vi "温度湿度监测界面.vi"() -> ()   [LabVIEW 2016, in "环境动力监测库.lvlib"]
panel:
  out "x+1":u32
  in  "解除告警":bool
  out "告警内容":string
  in  "高温告警启用":bool
  out "湿度显示":dbl=21.0 format="%.2f %%"
  out "湿度":dbl(graph)
  out "温度显示":dbl=21.0 format="%.2f ℃"
  out "温度":dbl(graph)
  in  "湿度下限告警点":dbl
  in  "湿度上限告警点":dbl
  in  "室温下限告警点":dbl
  in  "室温上限告警点":dbl
  # "温湿度监测"
  # "%"
  # "℃"
  # "%"
  # "℃"
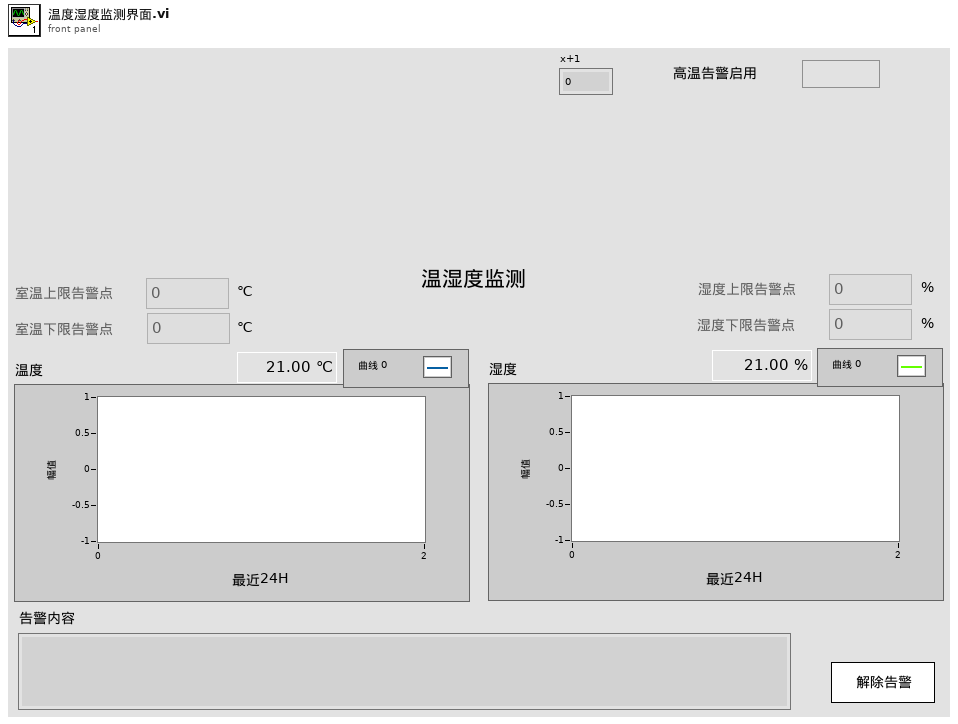
[diagram p1: front panel]
types:
  T1 = enum16{"报警状态监测", "报警确认", "仪器断电", "市电断电", "工控机关机", "取消告警", "结束"}
  T2 = cluster{"漏水监测输出":cluster{"漏水监测告警":bool, "告警内容":string}, "门禁监测输出":cluster{"门禁监测告警":bool, "告警内容":string}, "门禁监测输出2":cluster{"门禁监测告警":bool, "告警内容":string}, "温湿度监测输出":cluster{"温湿度监测告警":bool, "告警内容":string}, "烟雾监测输出":cluster{"烟雾监测告警":bool, "告警内容":string}, "空调监测输出":cluster{"空调监测告警":bool, "告警内容":string}, "自动重合闸输出":cluster{"自动重合闸告警":bool, "告警内容":string}, "红外入侵输出":cluster{"红外入侵告警":bool, "告警内容":string}, "振动输出":cluster{"振动告警":bool, "告警内容":string}, "UPS输出":cluster{"UPS告警":bool, "告警内容":string}, "蓄电池输出":cluster{"蓄电池告警":bool, "告警内容":string}, "蓄电池输出2":cluster{"蓄电池告警":bool, "告警内容":string}, "GPS输出":cluster{"定位告警":bool, "告警内容":string}, "北斗输出":cluster{"定位告警":bool, "告警内容":string}, "气象输出":cluster{"气象告警":bool, "告警内容":string}}
  T3 = cluster{"漏水监测配置":cluster{"监测项描述:输出":string, "端口:":enum16{"AI0", "AI1", "AI2", "AI3", "AI4", "DI0", "DI1", "DI2", "DI3", "DI4", "DO0", "DO1", "DO2", "DO3", "DO4", "X0", "X1", "X2", "X3", "X4", "X5", "X6", "X7", "X8", "X9", "X10", "X11", "X12", "X13", "X14", "X15", "X16", "X17", "X18", "X19", "X20", "X21", "X22", "X23"}, "告警参数:":enum32{"禁用告警", "闭合告警", "断开告警"}, "传感器型号:":enum16{"PLC", "ZLAN", "ART"}, "声光告警启用":bool}, "门禁开关监测配置":cluster{"监测项描述:输出":string, "端口:":enum16{"AI0", "AI1", "AI2", "AI3", "AI4", "DI0", "DI1", "DI2", "DI3", "DI4", "DO0", "DO1", "DO2", "DO3", "DO4", "X0", "X1", "X2", "X3", "X4", "X5", "X6", "X7", "X8", "X9", "X10", "X11", "X12", "X13", "X14", "X15", "X16", "X17", "X18", "X19", "X20", "X21", "X22", "X23"}, "告警参数:":enum32{"禁用告警", "闭合告警", "断开告警"}, "传感器型号:":enum16{"PLC", "ZLAN", "ART"}, "声光告警启用":bool}, "门禁开关监测配置2":cluster{"监测项描述:输出":string, "端口:":enum16{"AI0", "AI1", "AI2", "AI3", "AI4", "DI0", "DI1", "DI2", "DI3", "DI4", "DO0", "DO1", "DO2", "DO3", "DO4", "X0", "X1", "X2", "X3", "X4", "X5", "X6", "X7", "X8", "X9", "X10", "X11", "X12", "X13", "X14", "X15", "X16", "X17", "X18", "X19", "X20", "X21", "X22", "X23"}, "告警参数:":enum32{"禁用告警", "闭合告警", "断开告警"}, "传感器型号:":enum16{"PLC", "ZLAN", "ART"}, "声光告警启用":bool}, "温湿度监测配置":cluster{"监测项描述:输出":string, "端口:":enum16{"AI0", "AI1", "AI2", "AI3", "AI4", "DI0", "DI1", "DI2", "DI3", "DI4", "DO0", "DO1", "DO2", "DO3", "DO4", "X0", "X1", "X2", "X3", "X4", "X5", "X6", "X7", "X8", "X9", "X10", "X11", "X12", "X13", "X14", "X15", "X16", "X17", "X18", "X19", "X20", "X21", "X22", "X23"}, "告警参数:":enum32{"禁用告警", "闭合告警", "断开告警"}, "传感器型号:":enum16{"PLC", "ZLAN", "ART"}, "声光告警启用":bool}, "烟雾监测配置":cluster{"监测项描述:输出":string, "端口:":enum16{"AI0", "AI1", "AI2", "AI3", "AI4", "DI0", "DI1", "DI2", "DI3", "DI4", "DO0", "DO1", "DO2", "DO3", "DO4", "X0", "X1", "X2", "X3", "X4", "X5", "X6", "X7", "X8", "X9", "X10", "X11", "X12", "X13", "X14", "X15", "X16", "X17", "X18", "X19", "X20", "X21", "X22", "X23"}, "告警参数:":enum32{"禁用告警", "闭合告警", "断开告警"}, "传感器型号:":enum16{"PLC", "ZLAN", "ART"}, "声光告警启用":bool}, "冰箱监测配置":cluster{"监测项描述:输出":string, "端口:":enum16{"AI0", "AI1", "AI2", "AI3", "AI4", "DI0", "DI1", "DI2", "DI3", "DI4", "DO0", "DO1", "DO2", "DO3", "DO4", "X0", "X1", "X2", "X3", "X4", "X5", "X6", "X7", "X8", "X9", "X10", "X11", "X12", "X13", "X14", "X15", "X16", "X17", "X18", "X19", "X20", "X21", "X22", "X23"}, "告警参数:":enum32{"禁用告警", "闭合告警", "断开告警"}, "传感器型号:":enum16{"PLC", "ZLAN", "ART"}, "声光告警启用":bool}, "排气扇监测配置":cluster{"监测项描述:输出":string, "端口:":enum16{"AI0", "AI1", "AI2", "AI3", "AI4", "DI0", "DI1", "DI2", "DI3", "DI4", "DO0", "DO1", "DO2", "DO3", "DO4", "X0", "X1", "X2", "X3", "X4", "X5", "X6", "X7", "X8", "X9", "X10", "X11", "X12", "X13", "X14", "X15", "X16", "X17", "X18", "X19", "X20", "X21", "X22", "X23"}, "告警参数:":enum32{"禁用告警", "闭合告警", "断开告警"}, "传感器型号:":enum16{"PLC", "ZLAN", "ART"}, "声光告警启用":bool}, "红外入侵监测配置":cluster{"监测项描述:输出":string, "端口:":enum16{"AI0", "AI1", "AI2", "AI3", "AI4", "DI0", "DI1", "DI2", "DI3", "DI4", "DO0", "DO1", "DO2", "DO3", "DO4", "X0", "X1", "X2", "X3", "X4", "X5", "X6", "X7", "X8", "X9", "X10", "X11", "X12", "X13", "X14", "X15", "X16", "X17", "X18", "X19", "X20", "X21", "X22", "X23"}, "告警参数:":enum32{"禁用告警", "闭合告警", "断开告警"}, "传感器型号:":enum16{"PLC", "ZLAN", "ART"}, "声光告警启用":bool}, "振动监测配置":cluster{"监测项描述:输出":string, "端口:":enum16{"AI0", "AI1", "AI2", "AI3", "AI4", "DI0", "DI1", "DI2", "DI3", "DI4", "DO0", "DO1", "DO2", "DO3", "DO4", "X0", "X1", "X2", "X3", "X4", "X5", "X6", "X7", "X8", "X9", "X10", "X11", "X12", "X13", "X14", "X15", "X16", "X17", "X18", "X19", "X20", "X21", "X22", "X23"}, "告警参数:":enum32{"禁用告警", "闭合告警", "断开告警"}, "传感器型号:":enum16{"PLC", "ZLAN", "ART"}, "声光告警启用":bool}}
  T4 = cluster{"监测项描述:输出":string, "端口:":enum16{"AI0", "AI1", "AI2", "AI3", "AI4", "DI0", "DI1", "DI2", "DI3", "DI4", "DO0", "DO1", "DO2", "DO3", "DO4", "X0", "X1", "X2", "X3", "X4", "X5", "X6", "X7", "X8", "X9", "X10", "X11", "X12", "X13", "X14", "X15", "X16", "X17", "X18", "X19", "X20", "X21", "X22", "X23"}, "告警参数:":enum32{"禁用告警", "闭合告警", "断开告警"}, "传感器型号:":enum16{"PLC", "ZLAN", "ART"}, "声光告警启用":bool}
  T5 = enum16{"AI0", "AI1", "AI2", "AI3", "AI4", "DI0", "DI1", "DI2", "DI3", "DI4", "DO0", "DO1", "DO2", "DO3", "DO4", "X0", "X1", "X2", "X3", "X4", "X5", "X6", "X7", "X8", "X9", "X10", "X11", "X12", "X13", "X14", "X15", "X16", "X17", "X18", "X19", "X20", "X21", "X22", "X23"}
  T6 = cluster{"市电监测":bool, "用水量监测":bool, "烟雾监测":bool, "温度湿度":bool, "振动监测":bool, "红外入侵监测":bool, "漏水监测":bool, "门禁开关监测":bool, "门禁开关监测2":bool, "视频监测":bool, "UPS监测":bool, "空调监测":bool, "冰箱监测":bool, "排气扇监测":bool, "蓄电池监测":bool, "蓄电池监测2":bool, "GPS监测":bool, "北斗监测":bool, "气象监测":bool, "智能门禁监测":bool}
  T7 = cluster{"状态":cluster{"R0":i16, "R1":i16, "R2":i16, "R3":i16, "R4":i16, "R5":i16, "R6":i16, "R7":i16, "R8":i16, "R9":i16, "R10":i16, "R11":i16, "R12":i16, "R13":i16, "R14":i16, "R15":i16, "R16":i16, "R17":i16, "R18":i16, "R19":i16, "R20":i16, "R21":i16, "R22":i16, "R23":i16, "R24":i16, "R25":i16, "R26":i16, "R27":i16, "R28":i16, "R29":i16, "R30":i16, "R31":i16, "R32":i16, "R33":i16, "R34":i16, "R35":i16, "R36":i16, "R37":i16, "R38":i16, "R39":i16}, "输入状态":bool[], "输出状态":bool[], "参数设置":cluster{"R100":i16, "R101":i16, "R102":i16, "R103":i16, "R104":i16, "R105":i16, "R106":i16, "R107":i16, "R108":i16, "R109":i16, "R110":i16, "R111":i16, "R112":i16, "R113":i16, "R114":i16, "R115":i16, "R116":i16, "R117":i16, "R118":i16, "R119":i16, "R120":i16, "R121":i16, "R122":i16, "R123":i16}, "转换值":cluster{"AD0":sgl, "AD1":sgl, "AD2":sgl, "AD3":sgl, "AD4":sgl, "AD5":sgl}}
  T8 = cluster{"型号选择":enum16{"黑盾", "英维克", "仁科测控RS-KTC-N01"}, "MB session in":refnum<class "MB_Master.lvclass">, "英维克空调寄存器":u16[], "通讯状态":bool, "PORT":string, "IP":string, "Slave ID ":u8, "Serial Config":cluster{"baud rate (bps)":u32, "stop bits":u16, "parity":u16, "flow control":u16, "timeout":u32, "retries":i32}, "VISA Resource":refnum<visa-resource-name>, "MB通信方式选择":enum16{"串口", "TCP"}}
  T9 = cluster{"温湿度解析":cluster{"湿度":dbl, "温度":dbl}, "传感器状态输出":cluster{"第一路电流A":u16, "第二路电流A":u16, "空调控制模式":enum16{"远程", "自动"}, "蜂鸣器和继电器报警输出状态":enum16{"正常", "报警"}, "秒数高16位":u16, "秒数低16位":u16}, "告警状态":cluster{"第一路开关机失败":bool, "第二路开关机失败":bool, "温度超上限报警":bool, "温度超下限报警":bool}, "运行状态":cluster{"第一路空调运行状态":enum16{"停止", "制冷", "制热", "未知"}, "第二路空调运行状态":enum16{"停止", "制冷", "制热", "未知"}}}
  T10 = cluster{"状态":cluster{"R0":i16, "R1":i16, "R2":i16, "R3":i16, "R4":i16, "R5":i16, "R6":i16, "R7":i16, "R8":i16, "R9":i16, "R10":i16, "R11":i16, "R12":i16, "R13":i16, "R14":i16, "R15":i16, "R16":i16, "R17":i16, "R18":i16, "R19":i16, "R20":i16, "R21":i16, "R22":i16, "R23":i16, "R24":i16, "R25":i16, "R26":i16, "R27":i16, "R28":i16, "R29":i16, "R30":i16, "R31":i16, "R32":i16, "R33":i16, "R34":i16, "R35":i16, "R36":i16, "R37":i16, "R38":i16, "R39":i16, "R40":i16, "R41":i16, "R42":i16, "R43":i16, "R44":i16, "R45":i16, "R46":i16, "R47":i16, "R48":i16, "R49":i16, "R50":i16, "R51":i16, "R52":i16, "R53":i16, "R54":i16, "R55":i16, "R56":i16, "R57":i16, "R58":i16, "R59":i16, "R60":i16, "R61":i16, "R62":i16, "R63":i16, "R64":i16, "R65":i16, "R66":i16, "R67":i16, "R68":i16, "R69":i16}, "输入状态":bool[], "输出状态":bool[], "报警簇":bool[], "参数设置":cluster{"R100":i16, "R101":i16, "R102":i16, "R103":i16, "R104":i16, "R105":i16, "R106":i16, "R107":i16, "R108":i16, "R109":i16, "R110":i16, "R111":i16, "R112":i16, "R113":i16, "R114":i16, "R115":i16, "R116":i16, "R117":i16, "R118":i16, "R119":i16, "R120":i16, "R121":i16, "R122":i16, "R123":i16, "R124":i16}, "转换值":cluster{"AD0":sgl, "AD1":sgl, "AD2":sgl, "AD3":sgl, "AD4":sgl, "AD5":sgl}, "看门狗启用":bool, "氨氮模块名称":string, "总磷模块名称":string, "采配水模块类型":enum16{"V1", "V2", "V3", "V4", "室内V1", "室内V2"}}
  T11 = cluster{"AD0":dbl, "AD1":dbl, "AD2":dbl, "AD3":dbl, "AD4":dbl, "AD5":dbl, "AD6":dbl, "AD7":dbl}
  T12 = cluster{"命令":string, cluster{"starting address":u16, "holding register value":u16}}
  T13 = cluster{"温湿度":cluster{"状态":bool, "温度:":sgl, "湿度:":sgl, "详情  ":bool}, "空调":cluster{"状态":bool, "机柜温度:":sgl, "压缩机:":enum16{"停止", "运行"}, "电加热:":enum16{"停止", "运行"}, "详情  ":bool}, "排气扇":cluster{"排气扇":bool, "详情  ":bool}, "冰箱":cluster{"冰箱":bool, "详情  ":bool}}
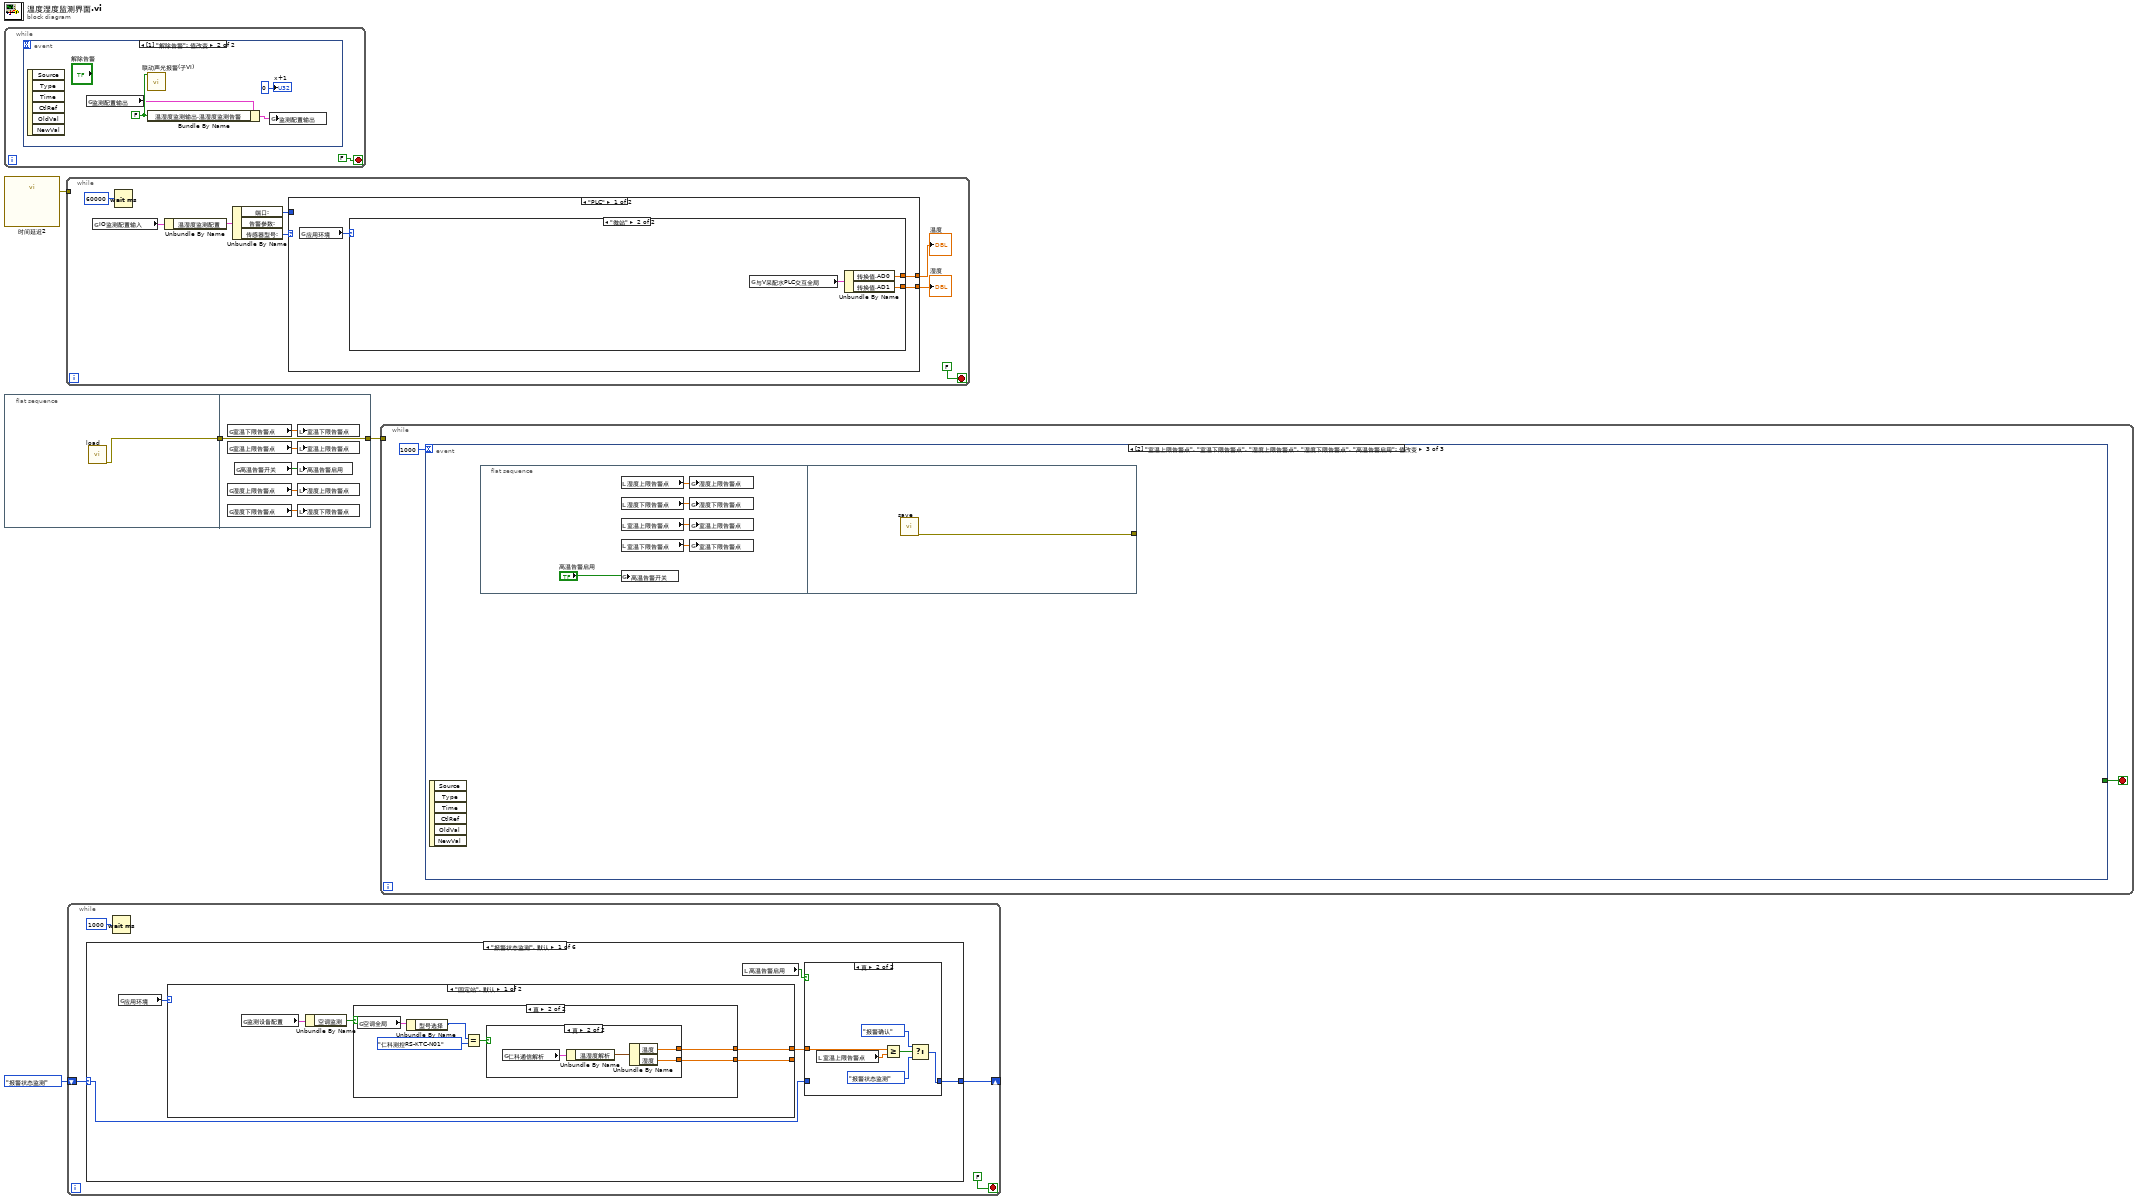
[diagram p0: block diagram]
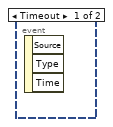
[diagram p2: hidden frame]
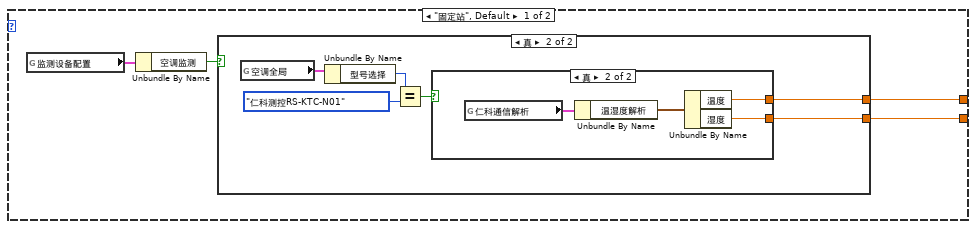
[diagram p3: hidden frame]
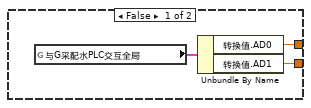
[diagram p4: hidden frame]
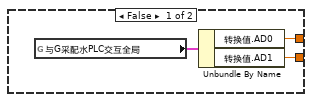
[diagram p5: hidden frame]
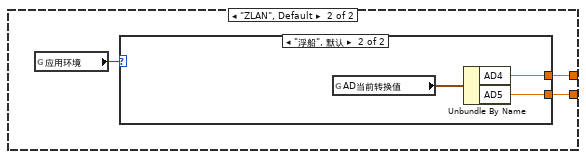
[diagram p6: hidden frame]
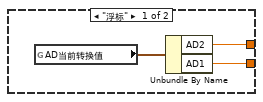
[diagram p7: hidden frame]
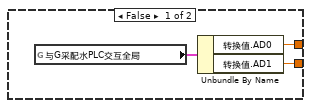
[diagram p8: hidden frame]
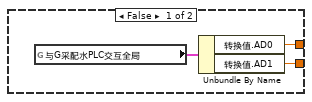
[diagram p9: hidden frame]
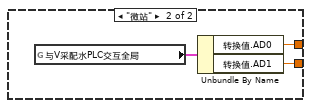
[diagram p10: hidden frame]
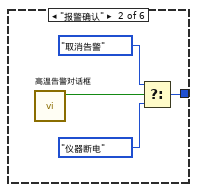
[diagram p12: hidden frame]
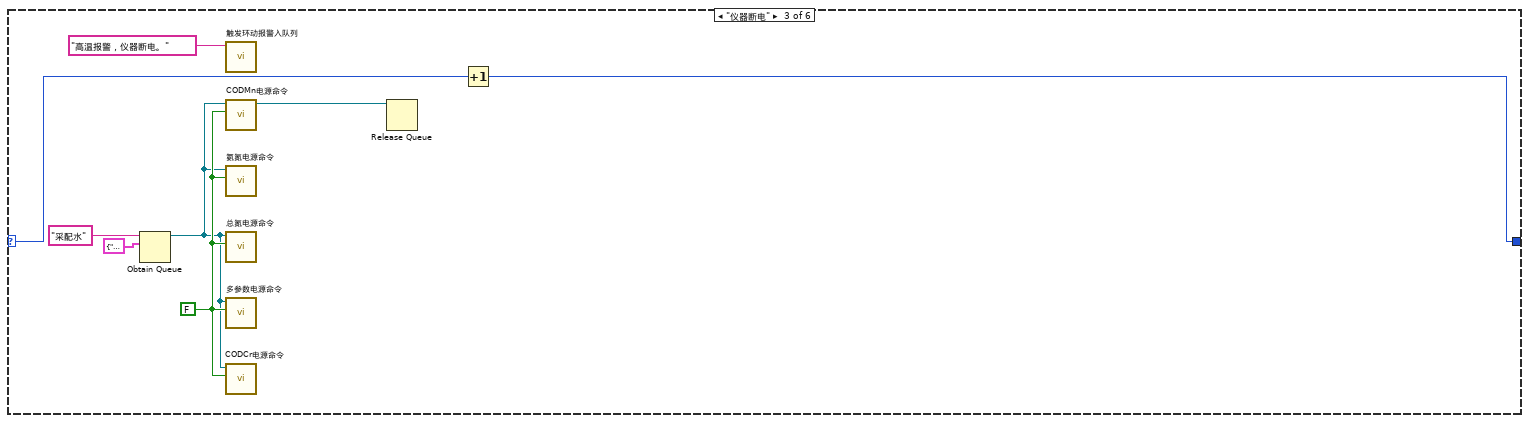
[diagram p13: hidden frame]
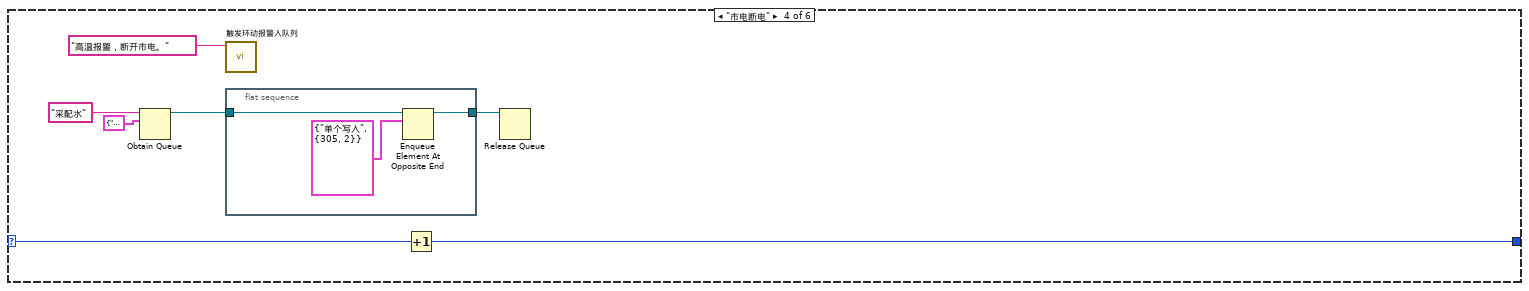
[diagram p14: hidden frame]
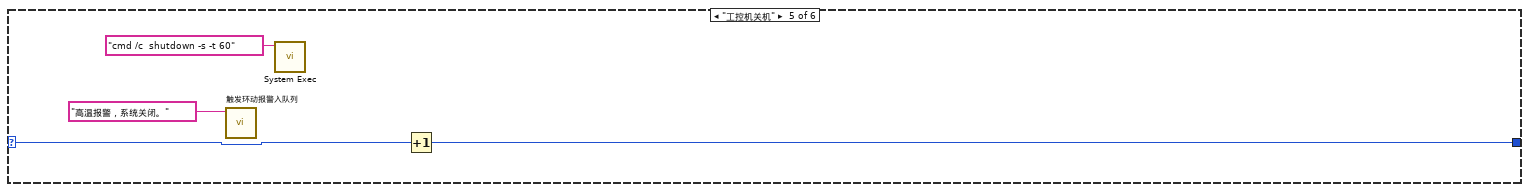
[diagram p15: hidden frame]
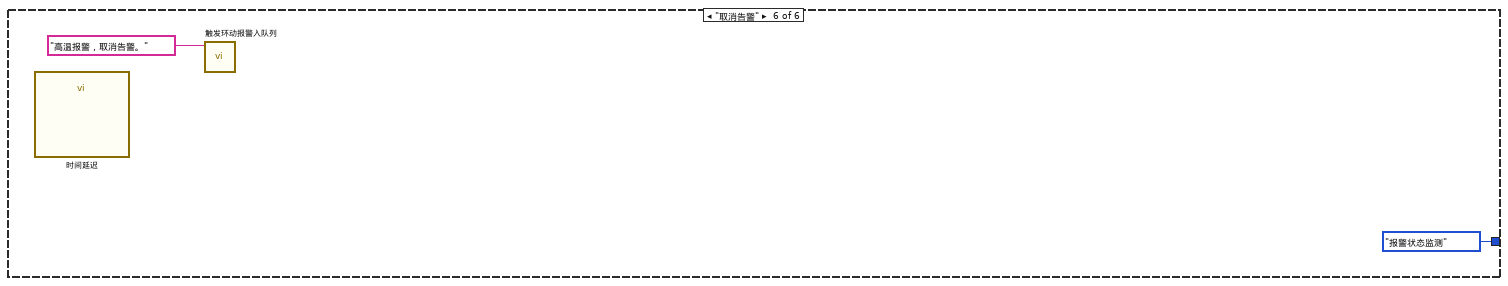
[diagram p16: hidden frame]
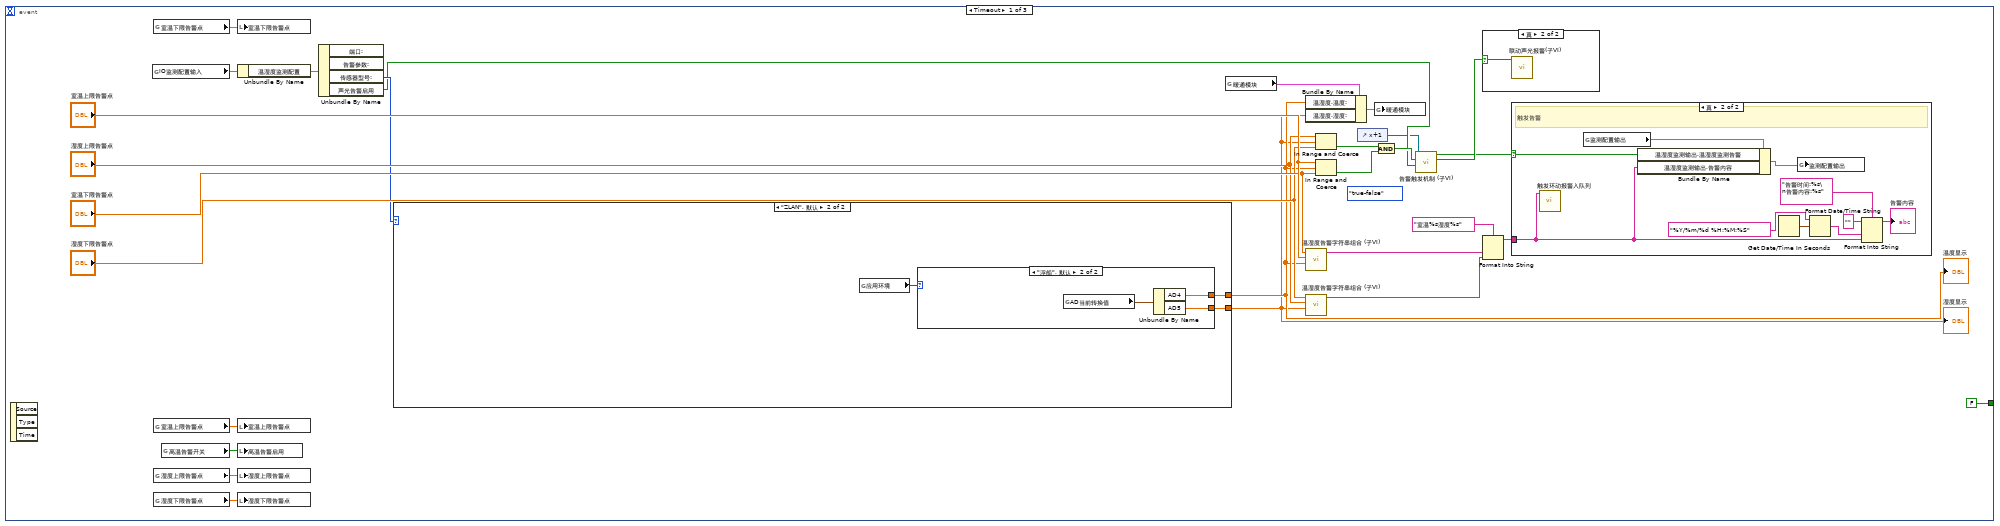
[diagram p17: hidden frame]
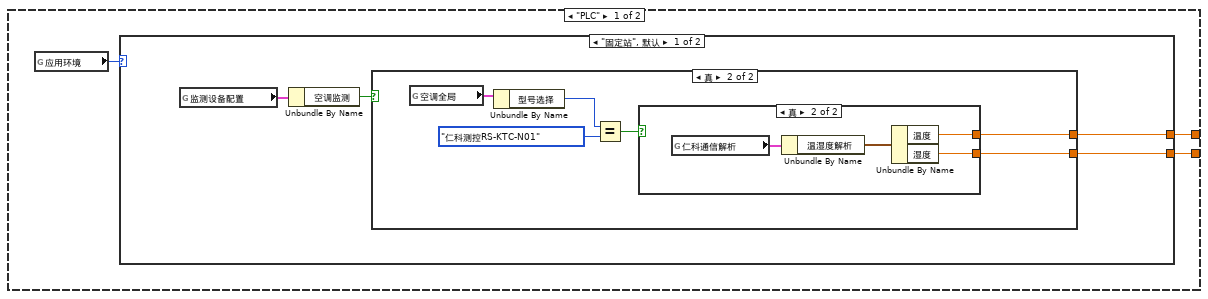
[diagram p19: hidden frame]
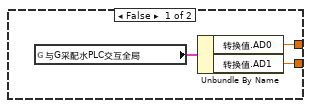
[diagram p20: hidden frame]
diagram:
  n1 = while {
    stop <- FALSE stop-if-true
    n2 = event shown="[1] \"解除告警\": 值改变" {
      selector: _ -> [_ _]
      dyn-events: _ -> [_ _]
      timeout: _ -> [_ _]
      event Timeout {
        n3 = event-data() -> ()  [unwired: 1 in, 3 out]
      }
      event "解除告警": Value Change {
        w9 = FALSE
        n4 = event-data() -> ()  [unwired: 1 in, 6 out]
        n5 = global read "内部交互全局变量.vi" "监测配置输出"() -> (w7:T2)
        n6 = call "联动声光报警(子VI).vi"("布尔"=w9) -> ()  [unwired: 11 in]
        n7 = Bundle By Name(cluster=w7, "温湿度监测输出.温湿度监测告警"=w9) -> (w6:T2)
        n8 = global write "内部交互全局变量.vi" "监测配置输出"(w6) -> ()
        "x+1" <- u32 0 ("x+1")
      }
    }
  }
  n9 = call "时间延迟2"() -> ("error out"=w1:errorcluster)  [unwired: 11 in]
  n10 = flat-sequence {
    tunnel: [w10] -> w4
    tunnel: [w16] -> w3
    tunnel: w4 -> [w16]
    frame #0 {
      n11 = call "load.vi"() -> ("error out"=w10:errorcluster)  [unwired: 11 in]
    }
    frame #1 {
      n12 = global read "断电保存全局变量.vi" "室温下限告警点"() -> (w15:dbl)
      n13 = global read "断电保存全局变量.vi" "室温上限告警点"() -> (w14:dbl)
      n14 = global read "断电保存全局变量.vi" "湿度上限告警点"() -> (w12:dbl)
      n15 = global read "断电保存全局变量.vi" "湿度下限告警点"() -> (w13:dbl)
      n16 = global read "断电保存全局变量.vi" "高温告警开关"() -> (w11:bool)
      n17 = local write "室温下限告警点"(w15) -> ()
      n18 = local write "室温上限告警点"(w14) -> ()
      n19 = local write "高温告警启用"(w11) -> ()
      n20 = local write "湿度上限告警点"(w12) -> ()
      n21 = local write "湿度下限告警点"(w13) -> ()
    }
  }
  n22 = while {
    tunnel: w1 -> [_]
    stop <- FALSE stop-if-true
    n23 = global read "断电保存全局变量.vi" "IO监测配置输入"() -> (w17:T3)
    n24 = Wait (ms)(milliseconds to wait=u32 60000 ("等待时间（毫秒）")) -> ()  [unwired: 1 out]
    n25 = Unbundle By Name(w17) -> ("温湿度监测配置"=w22:T4)
    n26 = Unbundle By Name(w22) -> ("端口:"=w20:T5, "传感器型号:"=w21:enum16{"PLC", "ZLAN", "ART"})  [unwired: 1 out]
    n27 = case shown="\"PLC\"" w21 {
      tunnel: w20 -> [_ _]
      tunnel: [w26 w52] -> w19
      tunnel: [w25 w51] -> w18
      frame "PLC" {
        n28 = global read "外部交互全局变量.vi" "应用环境"() -> (w27:enum16{"固定站", "微站", "浮标", "浮船"})
        n29 = case shown="\"微站\"" w27 {
          tunnel: [w29 w49] -> w26
          tunnel: [w28 w48] -> w25
          frame "固定站", Default {
            n30 = global read "断电保存全局变量.vi" "监测设备配置"() -> (w30:T6)
            n31 = Unbundle By Name(w30) -> ("空调监测"=w31:bool)
            n32 = case shown="真" w31 {
              tunnel: [w33 w38] -> w29
              tunnel: [w32 w37] -> w28
              frame False {
                n33 = global read "外部交互全局变量.vi" "与G采配水PLC交互全局"() -> (w34:T7)
                n34 = Unbundle By Name(w34) -> ("转换值.AD0"=w33:sgl, "转换值.AD1"=w32:sgl)
              }
              frame True {
                n35 = global read "断电保存全局变量.vi" "空调全局"() -> (w36:T8)
                n36 = Unbundle By Name(w36) -> ("型号选择"=w35:enum16{"黑盾", "英维克", "仁科测控RS-KTC-N01"})
                n37 = Equal?(x=w35, y=enum16{"黑盾", "英维克", "仁科测控RS-KTC-N01"}."仁科测控RS-KTC-N01") -> (x = y?=w39:bool)
                n38 = case shown="真" w39 {
                  tunnel: [w42 w45] -> w38
                  tunnel: [w41 w44] -> w37
                  frame False {
                    n39 = global read "外部交互全局变量.vi" "与G采配水PLC交互全局"() -> (w43:T7)
                    n40 = Unbundle By Name(w43) -> ("转换值.AD0"=w42:sgl, "转换值.AD1"=w41:sgl)
                  }
                  frame True {
                    n41 = global read "内部交互全局变量.vi" "仁科通信解析"() -> (w46:T9)
                    n42 = Unbundle By Name(w46) -> ("温湿度解析"=w47:cluster{"湿度":dbl, "温度":dbl})
                    n43 = Unbundle By Name(w47) -> ("温度"=w45:dbl, "湿度"=w44:dbl)
                  }
                }
              }
            }
          }
          frame "微站" {
            n44 = global read "外部交互全局变量.vi" "与V采配水PLC交互全局"() -> (w50:T10)
            n45 = Unbundle By Name(w50) -> ("转换值.AD0"=w49:sgl, "转换值.AD1"=w48:sgl)
          }
        }
      }
      frame "ZLAN", Default {
        n46 = global read "外部交互全局变量.vi" "应用环境"() -> (w53:enum16{"固定站", "微站", "浮标", "浮船"})
        n47 = case shown="\"浮船\", 默认" w53 {
          tunnel: [w56 w58] -> w52
          tunnel: [w55 w57] -> w51
          frame "浮标" {
            n48 = global read "断电保存全局变量.vi" "AD当前转换值"() -> (w54:T11)
            n49 = Unbundle By Name(w54) -> ("AD2"=w56:dbl, "AD1"=w55:dbl)
          }
          frame "浮船", Default {
            n50 = global read "断电保存全局变量.vi" "AD当前转换值"() -> (w59:T11)
            n51 = Unbundle By Name(w59) -> ("AD4"=w58:dbl, "AD5"=w57:dbl)
          }
        }
      }
    }
    "温度" <- w19
    "湿度" <- w18
  }
  n52 = while {
    shift-right: [w63] -> _
    shift-left: T1."报警状态监测" ("枚举") -> [w62]
    stop <- FALSE stop-if-true
    n53 = case shown="\"报警状态监测\", 默认" w62 {
      selector: w62 -> [w66 _ w109 w112 w123 _]
      tunnel: [w68 w99 w108 w111 w122 T1."报警状态监测" ("枚举")] -> w63
      frame "报警状态监测", Default {
        n54 = global read "外部交互全局变量.vi" "应用环境"() -> (w65:enum16{"固定站", "微站", "浮标", "浮船"})
        n55 = case shown="\"固定站\", 默认" w65 {
          tunnel: [w70 w90] -> w64
          tunnel: [w69 w89] -> _
          frame "固定站", Default {
            n56 = global read "断电保存全局变量.vi" "监测设备配置"() -> (w71:T6)
            n57 = Unbundle By Name(w71) -> ("空调监测"=w72:bool)
            n58 = case shown="真" w72 {
              tunnel: [w74 w79] -> w70
              tunnel: [w73 w78] -> w69
              frame False {
                n59 = global read "外部交互全局变量.vi" "与G采配水PLC交互全局"() -> (w75:T7)
                n60 = Unbundle By Name(w75) -> ("转换值.AD0"=w74:sgl, "转换值.AD1"=w73:sgl)
              }
              frame True {
                n61 = global read "断电保存全局变量.vi" "空调全局"() -> (w77:T8)
                n62 = Unbundle By Name(w77) -> ("型号选择"=w76:enum16{"黑盾", "英维克", "仁科测控RS-KTC-N01"})
                n63 = Equal?(x=w76, y=enum16{"黑盾", "英维克", "仁科测控RS-KTC-N01"}."仁科测控RS-KTC-N01") -> (x = y?=w80:bool)
                n64 = case shown="真" w80 {
                  tunnel: [w83 w86] -> w79
                  tunnel: [w82 w85] -> w78
                  frame False {
                    n65 = global read "外部交互全局变量.vi" "与G采配水PLC交互全局"() -> (w84:T7)
                    n66 = Unbundle By Name(w84) -> ("转换值.AD0"=w83:sgl, "转换值.AD1"=w82:sgl)
                  }
                  frame True {
                    n67 = global read "内部交互全局变量.vi" "仁科通信解析"() -> (w87:T9)
                    n68 = Unbundle By Name(w87) -> ("温湿度解析"=w88:cluster{"湿度":dbl, "温度":dbl})
                    n69 = Unbundle By Name(w88) -> ("温度"=w86:dbl, "湿度"=w85:dbl)
                  }
                }
              }
            }
          }
          frame "微站" {
            n70 = global read "外部交互全局变量.vi" "与V采配水PLC交互全局"() -> (w91:T10)
            n71 = Unbundle By Name(w91) -> ("转换值.AD0"=w90:sgl, "转换值.AD1"=w89:sgl)
          }
        }
        n72 = local read "高温告警启用"() -> (w67:bool)
        n73 = case shown="真" w67 {
          tunnel: [w92 w94] -> w68
          tunnel: w66 -> [w92 _]
          tunnel: w64 -> [_ w93]
          frame False {
          }
          frame True {
            n74 = local read "室温上限告警点"() -> (w98:dbl)
            n75 = Greater Or Equal?(x=w93, y=w98) -> (x >= y?=w97:bool)
            n76 = Select(t=T1."报警确认" ("枚举"), s=w97, f=T1."报警状态监测" ("枚举")) -> (s? t:f=w94:T1)
          }
        }
      }
      frame "报警确认" {
        n77 = call "高温告警对话框.vi"() -> ("T button?"=w100:bool)  [unwired: 11 in]
        n78 = Select(t=T1."取消告警" ("枚举"), s=w100, f=T1."仪器断电" ("枚举")) -> (s? t:f=w99:T1)
      }
      frame "仪器断电" {
        w107 = FALSE ("通电/断电")
        n79 = Obtain Queue(name (unnamed)="采配水" ("名称（未命名）"), element data type=cluster{"命令":string, "数据":variant} {"命令"="", "数据"=variant}) -> (queue out=w105:refnum<queue>)  [unwired: 3 in, 2 out]
        n80 = call "触发环动报警入队列.vi"("报警内容"="高温报警，仪器断电。" ("日志信息")) -> ()  [unwired: 11 in]
        n81 = call "CODMn电源命令.vi"("通电/断电"=w107, "队列"=w105) -> ("队列输出"=w106:refnum<queue>)  [unwired: 9 in]
        n82 = call "氨氮电源命令.vi"("通电/断电"=w107, "队列"=w105) -> ()  [unwired: 9 in, 1 out]
        n83 = call "总氮电源命令.vi"("通电/断电"=w107, "队列"=w105) -> ()  [unwired: 9 in, 1 out]
        n84 = call "多参数电源命令.vi"("通电/断电"=w107, "队列"=w105) -> ()  [unwired: 9 in, 1 out]
        n85 = call "CODCr电源命令.vi"("通电/断电"=w107, "队列"=w105) -> ()  [unwired: 9 in, 1 out]
        n86 = Release Queue(queue=w106) -> ()  [unwired: 2 in, 3 out]
        n87 = Increment(x=w109) -> (x+1=w108:T1)
      }
      frame "市电断电" {
        n88 = Obtain Queue(name (unnamed)="采配水" ("名称（未命名）"), element data type=cluster{"命令":string, "数据":variant} {"命令"="", "数据"=variant}) -> (queue out=w115:refnum<queue>)  [unwired: 3 in, 2 out]
        n89 = call "触发环动报警入队列.vi"("报警内容"="高温报警，断开市电。" ("日志信息")) -> ()  [unwired: 11 in]
        n90 = flat-sequence {
          tunnel: w115 -> [w119]
          tunnel: [w118] -> w114
          frame #0 {
            n91 = Enqueue Element At Opposite End(queue=w119, element=T12 {"命令"="单个写入", {"starting address"=305, "holding register value"=2}} ("元素")) -> (queue out=w118:refnum<queue>)  [unwired: 2 in, 2 out]
          }
        }
        n92 = Increment(x=w112) -> (x+1=w111:T1)
        n93 = Release Queue(queue=w114) -> ()  [unwired: 2 in, 3 out]
      }
      frame "工控机关机" {
        n94 = call "触发环动报警入队列.vi"("报警内容"="高温报警，系统关闭。" ("日志信息")) -> ()  [unwired: 11 in]
        n95 = call <vilib>:"System Exec.vi"("command line"="cmd /c  shutdown -s -t 60") -> ()  [unwired: 7 in, 4 out]
        n96 = Increment(x=w123) -> (x+1=w122:T1)
      }
      frame "取消告警" {
        n97 = call "时间延迟"() -> ()  [unwired: 11 in, 1 out]
        n98 = call "触发环动报警入队列.vi"("报警内容"="高温报警，取消告警。" ("日志信息")) -> ()  [unwired: 11 in]
      }
    }
    n99 = Wait (ms)(milliseconds to wait=u32 1000 ("等待时间（毫秒）")) -> ()  [unwired: 1 out]
  }
  n100 = while {
    tunnel: w3 -> [_]
    stop <- w128 stop-if-true
    n101 = event shown="[2] \"室温上限告警点\", \"室温下限告警点\", \"湿度上限告警点\", \"湿度下限告警点\", \"高温告警启用\": 值改变" {
      selector: _ -> [_ _ _]
      dyn-events: _ -> [_ _ _]
      timeout: 1000 -> [_ _ _]
      tunnel: [FALSE _ _] -> w128
      event Timeout {
        (unwired) enum16{"either", "false-true", "true-false"}."true-false" ("direction")
        n102 = event-data() -> ()  [unwired: 1 in, 3 out]
        n103 = global read "断电保存全局变量.vi" "IO监测配置输入"() -> (w144:T3)
        n104 = global read "断电保存全局变量.vi" "室温下限告警点"() -> (w138:dbl)
        n105 = global read "断电保存全局变量.vi" "室温上限告警点"() -> (w137:dbl)
        n106 = global read "断电保存全局变量.vi" "湿度上限告警点"() -> (w135:dbl)
        n107 = global read "断电保存全局变量.vi" "湿度下限告警点"() -> (w136:dbl)
        n108 = global read "断电保存全局变量.vi" "高温告警开关"() -> (w134:bool)
        n109 = local write "室温下限告警点"(w138) -> ()
        n110 = Unbundle By Name(w144) -> ("温湿度监测配置"=w154:T4)
        n111 = local write "室温上限告警点"(w137) -> ()
        n112 = local write "高温告警启用"(w134) -> ()
        n113 = local write "湿度上限告警点"(w135) -> ()
        n114 = local write "湿度下限告警点"(w136) -> ()
        n115 = Unbundle By Name(w154) -> ("传感器型号:"=w143:enum16{"PLC", "ZLAN", "ART"}, "声光告警启用"=w131:bool)  [unwired: 2 out]
        n116 = case shown="\"ZLAN\", 默认" w143 {
          tunnel: [w158 w185] -> w140
          tunnel: [w159 w184] -> w139
          frame "PLC" {
            n117 = global read "外部交互全局变量.vi" "应用环境"() -> (w160:enum16{"固定站", "微站", "浮标", "浮船"})
            n118 = case shown="\"固定站\", 默认" w160 {
              tunnel: [w162 w182] -> w158
              tunnel: [w161 w181] -> w159
              frame "固定站", Default {
                n119 = global read "断电保存全局变量.vi" "监测设备配置"() -> (w163:T6)
                n120 = Unbundle By Name(w163) -> ("空调监测"=w164:bool)
                n121 = case shown="真" w164 {
                  tunnel: [w166 w171] -> w162
                  tunnel: [w165 w170] -> w161
                  frame False {
                    n122 = global read "外部交互全局变量.vi" "与G采配水PLC交互全局"() -> (w167:T7)
                    n123 = Unbundle By Name(w167) -> ("转换值.AD0"=w166:sgl, "转换值.AD1"=w165:sgl)
                  }
                  frame True {
                    n124 = global read "断电保存全局变量.vi" "空调全局"() -> (w169:T8)
                    n125 = Unbundle By Name(w169) -> ("型号选择"=w168:enum16{"黑盾", "英维克", "仁科测控RS-KTC-N01"})
                    n126 = Equal?(x=w168, y=enum16{"黑盾", "英维克", "仁科测控RS-KTC-N01"}."仁科测控RS-KTC-N01") -> (x = y?=w172:bool)
                    n127 = case shown="真" w172 {
                      tunnel: [w175 w178] -> w171
                      tunnel: [w174 w177] -> w170
                      frame False {
                        n128 = global read "外部交互全局变量.vi" "与G采配水PLC交互全局"() -> (w176:T7)
                        n129 = Unbundle By Name(w176) -> ("转换值.AD0"=w175:sgl, "转换值.AD1"=w174:sgl)
                      }
                      frame True {
                        n130 = global read "内部交互全局变量.vi" "仁科通信解析"() -> (w179:T9)
                        n131 = Unbundle By Name(w179) -> ("温湿度解析"=w180:cluster{"湿度":dbl, "温度":dbl})
                        n132 = Unbundle By Name(w180) -> ("温度"=w178:dbl, "湿度"=w177:dbl)
                      }
                    }
                  }
                }
              }
              frame "微站" {
                n133 = global read "外部交互全局变量.vi" "与V采配水PLC交互全局"() -> (w183:T10)
                n134 = Unbundle By Name(w183) -> ("转换值.AD0"=w182:sgl, "转换值.AD1"=w181:sgl)
              }
            }
          }
          frame "ZLAN", Default {
            n135 = global read "外部交互全局变量.vi" "应用环境"() -> (w186:enum16{"固定站", "微站", "浮标", "浮船"})
            n136 = case shown="\"浮船\", 默认" w186 {
              tunnel: [w189 w191] -> w185
              tunnel: [w188 w190] -> w184
              frame "浮标" {
                n137 = global read "断电保存全局变量.vi" "AD当前转换值"() -> (w187:T11)
                n138 = Unbundle By Name(w187) -> ("AD2"=w189:dbl, "AD1"=w188:dbl)
              }
              frame "浮船", Default {
                n139 = global read "断电保存全局变量.vi" "AD当前转换值"() -> (w192:T11)
                n140 = Unbundle By Name(w192) -> ("AD4"=w191:dbl, "AD5"=w190:dbl)
              }
            }
          }
        }
        "温度显示" <- w140
        "湿度显示" <- w139
        n141 = global read "内部交互全局变量.vi" "暖通模块"() -> (w142:T13)
        n142 = Bundle By Name(cluster=w142, "温湿度.温度:"=w140, "温湿度.湿度:"=w139) -> (w141:T13)
        n143 = call "温湿度告警字符串组合 (子VI).vi"("AD01"=w140, "室温湿度上限告警点"="室温上限告警点", "室温湿度下限告警点"="室温下限告警点") -> ("字符串"=w147:string)  [unwired: 8 in]
        n144 = call "温湿度告警字符串组合 (子VI).vi"("AD01"=w139, "室温湿度上限告警点"="湿度上限告警点", "室温湿度下限告警点"="湿度下限告警点") -> ("字符串"=w146:string)  [unwired: 8 in]
        n145 = In Range and Coerce(upper limit="湿度上限告警点", x=w139, lower limit="湿度下限告警点") -> (In Range?=w155:bool)  [unwired: 1 out]
        n146 = In Range and Coerce(upper limit="室温上限告警点", x=w140, lower limit="室温下限告警点") -> (In Range?=w153:bool)  [unwired: 1 out]
        n147 = control-ref of="x+1"() -> (w129:refnum<vi>)
        n148 = global write "内部交互全局变量.vi" "暖通模块"(w141) -> ()
        n149 = And(x=w155, y=w153) -> (x .and. y?=w133:bool)
        n150 = call "告警触发机制 (子VI).vi"("声光告警启用"=w131, "状态输出"=w133, "Digital输入"=w129) -> ("声光告警"=w132:bool, "触发告警"=w130:bool)  [unwired: 7 in]
        n151 = case shown="真" w132 {
          selector: w132 -> [_ w157]
          frame False {
          }
          frame True {
            n152 = call "联动声光报警(子VI).vi"("布尔"=w157) -> ()  [unwired: 11 in]
          }
        }
        n153 = Format Into String(format string="室温%s湿度%s" ("格式字符串"), w147, w146) -> (resulting string=w145:string)  [unwired: 2 in, 1 out]
        n154 = case shown="真" w130 {
          selector: w130 -> [_ w202]
          tunnel: w145 -> [_ w195]
          frame False {
          }
          frame True {
            # "触发告警"
            n155 = call "触发环动报警入队列.vi"("报警内容"=w195) -> ()  [unwired: 11 in]
            n156 = global read "内部交互全局变量.vi" "监测配置输出"() -> (w194:T2)
            n157 = Bundle By Name(cluster=w194, "温湿度监测输出.温湿度监测告警"=w202, "温湿度监测输出.告警内容"=w195) -> (w193:T2)
            n158 = Get Date/Time In Seconds() -> (seconds since 1Jan1904=w198:timestamp)
            n159 = global write "内部交互全局变量.vi" "监测配置输出"(w193) -> ()
            n160 = Format Date/Time String(time format string (%c)="%Y/%m/%d %H:%M:%S" ("时间格式字符串(%c)"), seconds (now)=w198) -> (date/time string=w200:string)  [unwired: 1 in]
            n161 = Format Into String(format string="告警时间:%s\n告警内容:%s" ("格式字符串"), initial string="" ("初始字符串"), w200, w195) -> (resulting string=→"告警内容":string)  [unwired: 1 in, 1 out]
          }
        }
      }
      event "室温上限告警点", "室温下限告警点", "湿度上限告警点", "湿度下限告警点": Mouse Down {
        n162 = event-data() -> ("CtlRef"=w206:refnum<vi>)  [unwired: 1 in, 7 out]
        n163 = property class="DigNum (严格)"(reference=w206) -> (reference out=w204:refnum<vi>, "Value"=w205:dbl)  [unwired: 1 in, 1 out]
        n164 = call "数字键盘.vi"("OldNumber"=w205) -> ("NewNumber"=w203:sgl)
        n165 = property class="DigNum (严格)"(reference=w204, "Val(Sgnl)"=w203) -> ()  [unwired: 1 in, 2 out]
      }
      event "室温上限告警点", "室温下限告警点", "湿度上限告警点", "湿度下限告警点", "高温告警启用": Value Change {
        n166 = event-data() -> ()  [unwired: 1 in, 6 out]
        n167 = flat-sequence {
          tunnel: [w212] -> _
          frame #0 {
            n168 = local read "湿度上限告警点"() -> (w211:dbl)
            n169 = local read "湿度下限告警点"() -> (w210:dbl)
            n170 = local read "室温上限告警点"() -> (w209:dbl)
            n171 = local read "室温下限告警点"() -> (w208:dbl)
            n172 = global write "断电保存全局变量.vi" "高温告警开关"("高温告警启用") -> ()
            n173 = global write "断电保存全局变量.vi" "湿度上限告警点"(w211) -> ()
            n174 = global write "断电保存全局变量.vi" "湿度下限告警点"(w210) -> ()
            n175 = global write "断电保存全局变量.vi" "室温上限告警点"(w209) -> ()
            n176 = global write "断电保存全局变量.vi" "室温下限告警点"(w208) -> ()
          }
          frame #1 {
            n177 = call "save.vi"() -> ("error out"=w212:errorcluster)  [unwired: 11 in]
          }
        }
      }
    }
  }
